vi "G# - CreatingAndDestroyingObjectsSubClasses.vi"() -> ()   [LabVIEW 2020]
doc: "This example will show how to create and destroy an object by using subclasses.\nThe classes are created with different templates, but with the exact same methods setting both attributes according to controls. Notice the difference in how attributes are modified. Notice that inherited methods has been used and also how to modify a parent attribute inside a method is shown.\n\nThe G#Template performance is better than the G#BaseTemplateG3 when using the Data Value Reference structure.\n\nBy using the G# Debugger found in Tools->G# Debugger a text log can be followed showing how the objects were created and destroyed and if you run the example with highlight execution enabled, you could also monitor the attributes value change."
uses:
  MyG#G3SubTempl_class/MyG#G3SubTempl.lvclass
  MyG#SubClass_class/MyG#SubClass.lvclass
  vi.lib/addons/_AddQ/G#Object/G#Object.lvclass
panel:
  in  "increment both Attributes":dbl=3.0
  in  "increment only G#G3Templ Attribute":dbl=2.0
  in  "Initial Value G#G3Temp attributes":dbl=12.0
  in  "increment both Attributes":dbl=3.0
  in  "increment only G# Object Attribute":dbl=2.0
  in  "Inital Value G# attributes":dbl=12.0
  out "My G# Object Sub Attribute out":dbl
  out "My G#G3Templ Sub Attribute out":dbl
  out "My G#G3Templ Attribute out":dbl
  in  "error in (no error)":errorcluster
  out "# of objects killed":i32
  out "OK":bool
  out "My G# Object Attribute out":dbl
  out "error out":errorcluster
  # "This example will show how to create and destroy an object by using subclasses.\nThe classes are created with different templates, but with the exact same methods setting both attributes according to controls.\nNotice the difference in how attributes are modified. Notice that inherited methods has been used and also how to modify a parent attribute inside a method is shown.\n\nThe G#Template performance is better than the G#BaseTemplateG3 when using the Data Value Reference structure.\n\nBy using the G# Debugger found in Tools->G# Debugger a text log can be followed showing how the objects were created and destroyed and if you run the example\nwith highlight execution enabled, you could also monitor the attributes value change."
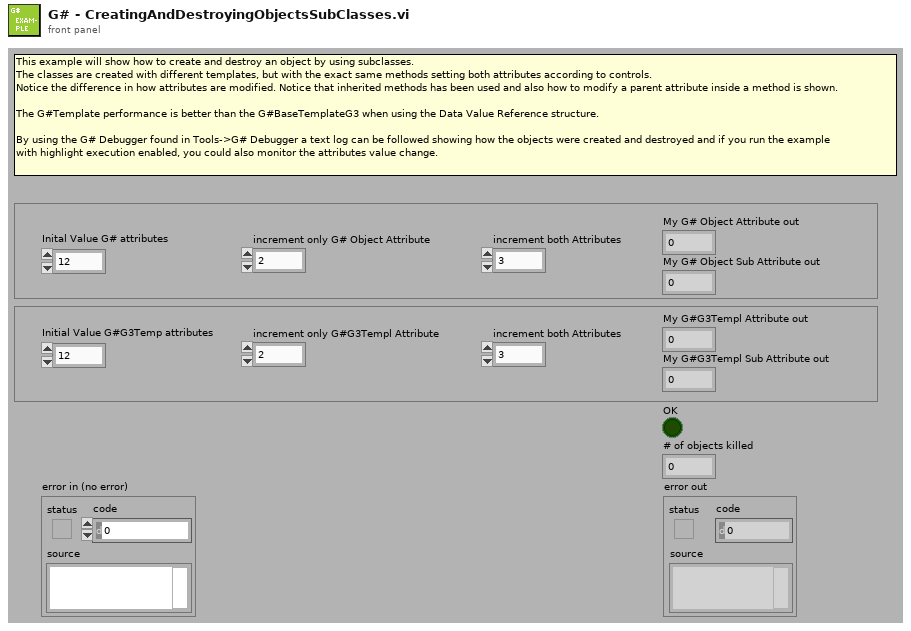
[diagram p1: front panel]
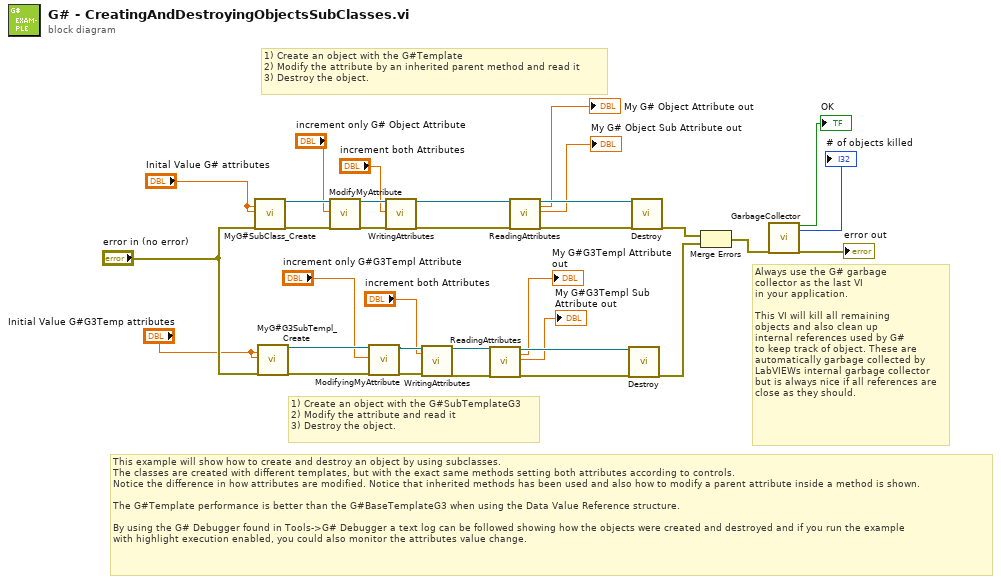
[diagram p0: block diagram]
diagram:
  # "This example will show how to create and destroy an object by using subclasses.\nThe classes are created with different templates, but with the exact same methods setting both attributes according to controls.\nNotice the difference in how attributes are modified. Notice that inherited methods has been used and also how to modify a parent attribute inside a method is shown.\n\nThe G#Template performance is better than the G#BaseTemplateG3 when using the Data Value Reference structure.\n\nBy using the G# Debugger found in Tools->G# Debugger a text log can be followed showing how the objects were created and destroyed and if you run the example\nwith highlight execution enabled, you could also monitor the attributes value change."
  # "Always use the G# garbage\ncollector as the last VI\nin your application.\n\nThis VI will kill all remaining\nobjects and also clean up\ninternal references used by G#\nto keep track of object. These are\nautomatically garbage collected by\nLabVIEWs internal garbage collector\nbut is always nice if all references are\nclose as they should."
  # "1) Create an object with the G#SubTemplateG3\n2) Modify the attribute and read it\n3) Destroy the object."
  # "1) Create an object with the G#Template\n2) Modify the attribute by an inherited parent method and read it\n3) Destroy the object."
  n1 = call "MyG#SubClass_Create.vi"("MySubAttribute"="Inital Value G# attributes", "MyAttribute"="Inital Value G# attributes", "error in (no error)"="error in (no error)") -> ("reference out"=w32:refnum<class "MyG#SubClass.lvclass">, "error out"=w33:errorcluster)  [unwired: 15 in]
  n2 = call "MyG#G3SubTempl_Create.vi"("MyAttribute"="Initial Value G#G3Temp attributes", "MySubAttribute"="Initial Value G#G3Temp attributes", "error in (no error)"="error in (no error)") -> ("reference out"=w28:refnum<class "MyG#G3SubTempl.lvclass">, "error out"=w29:errorcluster)  [unwired: 15 in]
  n3 = call-dynamic "ModifyMyAttribute.vi"("reference in"=w32, "increment"="increment only G# Object Attribute", "error in (no error)"=w33) -> ("reference out"=w8:refnum<class "MyG#SubClass.lvclass">, "error out"=w7:errorcluster)  [unwired: 15 in]
  n4 = call-dynamic "ModifyingMyAttribute.vi"("reference in"=w28, "increment"="increment only G#G3Templ Attribute", "error in (no error)"=w29) -> ("reference out"=w16:refnum<class "MyG#G3SubTempl.lvclass">, "error out"=w17:errorcluster)  [unwired: 15 in]
  n5 = call-dynamic "WritingAttributes.vi"("reference in"=w8, "increment"="increment both Attributes", "error in (no error)"=w7) -> ("reference out"=w5:refnum<class "MyG#SubClass.lvclass">, "error out"=w6:errorcluster)  [unwired: 15 in]
  n6 = call-dynamic "WritingAttributes.vi"("reference in"=w16, "increment"="increment both Attributes", "error in (no error)"=w17) -> ("reference out"=w14:refnum<class "MyG#G3SubTempl.lvclass">, "error out"=w13:errorcluster)  [unwired: 15 in]
  n7 = call-dynamic "ReadingAttributes.vi"("reference in"=w14, "error in (no error)"=w13) -> ("reference out"=w11:refnum<class "MyG#G3SubTempl.lvclass">, "Base class.MyAttribute"=→"My G#G3Templ Attribute out":dbl, "MySubAttribute"=→"My G#G3Templ Sub Attribute out":dbl, "error out"=w12:errorcluster)  [unwired: 14 in]
  n8 = call-dynamic "ReadingAttributes.vi"("reference in"=w5, "error in (no error)"=w6) -> ("reference out"=w31:refnum<class "MyG#SubClass.lvclass">, "MyAttribute"=→"My G# Object Attribute out":dbl, "MySubAttribute"=→"My G# Object Sub Attribute out":dbl, "error out"=w30:errorcluster)  [unwired: 14 in]
  n9 = call-dynamic "Destroy.vi"("reference in"=w11, "error in (no error)"=w12) -> ("error out"=w26:errorcluster)  [unwired: 16 in, 1 out]
  n10 = call-dynamic "Destroy.vi"("reference in"=w31, "error in (no error)"=w30) -> ("error out"=w27:errorcluster)  [unwired: 16 in, 1 out]
  n11 = Merge Errors(w27, w26) -> (w22:errorcluster)
  n12 = call "GarbageCollector.vi"("error in (no error)"=w22) -> ("OK"=→"OK":bool, "# of objects killed"=→"# of objects killed":i32, "error out"=→"error out":errorcluster)  [unwired: 16 in]
